vi "HFRR ADV v01.vi"() -> ()   [LabVIEW 2025] (continued)
            n2946 = case shown="False" w3205 {
              frame False {
                n2947 = disable-structure shown="Disabled" {
                  frame Disabled {
                    n2948 = stacked-sequence {
                      frame #0 {
                        n2949 = local write "RUN"(FALSE ("OK Button 2")) -> ()
                      }
                      frame #1 {
                      }
                    }
                  }
                  frame Enabled {
                  }
                }
              }
              frame True {
              }
            }
          }
        }
        n2950 = local read "Reset Graph"() -> (w3102:bool)
        n2951 = case shown="True" w3102 {
          selector: w3102 -> [_ w3119]
          frame False {
          }
          frame True {
            w3133 = 0.0 ("X Scale.Range:Maximum")
            n2952 = Not(x=w3119) -> (.not. x?=w3118:bool)
            n2953 = local write "Reset Graph"(w3118) -> ()
            n2954 = property on="Electrical Contact Resistance ( % )" class="WFChart (strict)"("XScale.Maximum"=600.0 ("X Scale.Range:Maximum"), "XScale.Minimum"=0.0 ("X Scale.Range:Minimum"), "YScale.Maximum"=100.0 ("Y Scale.Range:Maximum"), "YScale.Minimum"=0.0 ("Y Scale.Range:Minimum")) -> ()  [unwired: 2 in, 2 out]
            n2955 = property on="Frictional Force ( N )" class="WFChart (strict)"("XScale.Maximum"=600.0 ("X Scale.Range:Maximum"), "XScale.Minimum"=0.0 ("X Scale.Range:Minimum"), "YScale.Maximum"=100.0 ("Y Scale.Range:Maximum"), "YScale.Minimum"=0.0 ("Y Scale.Range:Minimum")) -> ()  [unwired: 2 in, 2 out]
            n2956 = property on="Temperature ( Deg C )" class="WFChart (strict)"("XScale.Maximum"=600.0 ("X Scale.Range:Maximum"), "XScale.Minimum"=0.0 ("X Scale.Range:Minimum"), "YScale.Maximum"=100.0 ("Y Scale.Range:Maximum"), "YScale.Minimum"=0.0 ("Y Scale.Range:Minimum")) -> ()  [unwired: 2 in, 2 out]
            n2957 = property on="Stroke ( mm )" class="WFChart (strict)"("XScale.Maximum"=600.0 ("X Scale.Range:Maximum"), "XScale.Minimum"=0.0 ("X Scale.Range:Minimum"), "YScale.Maximum"=100.0 ("Y Scale.Range:Maximum"), "YScale.Minimum"=0.0 ("Y Scale.Range:Minimum")) -> ()  [unwired: 2 in, 2 out]
            n2958 = property on="Coefficient of Friction" class="WFChart (strict)"("XScale.Maximum"=600.0 ("X Scale.Range:Maximum"), "XScale.Minimum"=0.0 ("X Scale.Range:Minimum"), "YScale.Maximum"=100.0 ("Y Scale.Range:Maximum"), "YScale.Minimum"=0.0 ("Y Scale.Range:Minimum")) -> ()  [unwired: 2 in, 2 out]
            n2959 = property on="Electrical Contact Resistance ( % )" class="WFChart (strict)"("XScale.Minimum"=0.0 ("X Scale.Range:Minimum"), "XScale.Maximum"=600.0 ("X Scale.Range:Maximum"), "YScale.Minimum"=0.0 ("Y Scale.Range:Minimum"), "YScale.Maximum"=100.0 ("Y Scale.Range:Maximum")) -> ()  [unwired: 2 in, 2 out]
            n2960 = property on="Temperature ( Deg C )" class="WFChart (strict)"("XScale.Minimum"=0.0 ("X Scale.Range:Minimum"), "XScale.Maximum"=600.0 ("X Scale.Range:Maximum"), "YScale.Minimum"=0.0 ("Y Scale.Range:Minimum"), "YScale.Maximum"=100.0 ("Y Scale.Range:Maximum")) -> ()  [unwired: 2 in, 2 out]
            n2961 = property on="Coefficient of Friction" class="WFChart (strict)"("XScale.Minimum"=0.0 ("X Scale.Range:Minimum"), "XScale.Maximum"=600.0 ("X Scale.Range:Maximum"), "YScale.Maximum"=1.0 ("X Scale.Range:Minimum"), "YScale.Minimum"=0.0 ("X Scale.Range:Minimum")) -> ()  [unwired: 2 in, 2 out]
            n2962 = property on="Frictional Force ( N )" class="WFChart (strict)"("XScale.Maximum"=600.0 ("X Scale.Range:Maximum"), "XScale.Minimum"=w3133, "YScale.Maximum"=10.0 ("Y Scale.Range:Maximum"), "YScale.Minimum"=w3133) -> ()  [unwired: 2 in, 2 out]
            n2963 = property on="Stroke ( mm )" class="WFChart (strict)"("XScale.Maximum"=600.0 ("X Scale.Range:Maximum"), "XScale.Minimum"=0.0 ("X Scale.Range:Minimum"), "YScale.Maximum"=100.0 ("Y Scale.Range:Maximum"), "YScale.Minimum"=0.0 ("Y Scale.Range:Minimum")) -> ()  [unwired: 2 in, 2 out]
          }
        }
      }
      frame "Compare Files" {
        # "Elapsed time\ncof\nstroke\nAir temp\nTemp\nHumidity"
        n2964 = case shown="True" "RSTV1 2" {
          frame False {
          }
          frame True {
            n2965 = property on="Humidity ( %RH )" class="XYGraph (strict)"("Y Scale.Display Format:Precision"=u8 0 ("Y Scale.Format & Precision:Precision")) -> ()  [unwired: 2 in, 2 out]
            n2966 = property on="Humidity ( %RH )" class="XYGraph (strict)"("X Scale.Range:Minimum"=0.0, "X Scale.Range:Maximum"=75.0, "Y Scale.Range:Minimum"=48.0, "Y Scale.Range:Maximum"=58.0) -> ()  [unwired: 2 in, 2 out]
          }
        }
        n2967 = case shown="True" "RST CP 2" {
          frame False {
          }
          frame True {
            n2968 = property on="XY Graph 13" class="XYGraph (strict)"("Y Scale.Display Format:Precision"=u8 0 ("Y Scale.Format & Precision:Precision")) -> ()  [unwired: 2 in, 2 out]
            n2969 = property on="XY Graph 13" class="XYGraph (strict)"("X Scale.Range:Minimum"=0.0, "X Scale.Range:Maximum"=75.0, "Y Scale.Range:Minimum"=0.0, "Y Scale.Range:Maximum"=100.0) -> ()  [unwired: 2 in, 2 out]
          }
        }
        n2970 = case shown="True" "RST CP" {
          frame False {
          }
          frame True {
            n2971 = property on="Sample Temperature ( °C )" class="XYGraph (strict)"("Y Scale.Display Format:Precision"=u8 2 ("Y Scale.Format & Precision:Precision")) -> ()  [unwired: 2 in, 2 out]
            n2972 = property on="Sample Temperature ( °C )" class="XYGraph (strict)"("X Scale.Range:Minimum"=0.0, "X Scale.Range:Maximum"=75.0, "Y Scale.Range:Minimum"=58.0, "Y Scale.Range:Maximum"=62.0) -> ()  [unwired: 2 in, 2 out]
          }
        }
        n2973 = case shown="True" "RSTV1 3" {
          frame False {
          }
          frame True {
            n2974 = property on="Air Temperature  ( °C )" class="XYGraph (strict)"("Y Scale.Display Format:Precision"=u8 2 ("Y Scale.Format & Precision:Precision")) -> ()  [unwired: 2 in, 2 out]
            n2975 = property on="Air Temperature  ( °C )" class="XYGraph (strict)"("X Scale.Range:Minimum"=0.0 ("Y Scale.Range:Minimum"), "X Scale.Range:Maximum"=75.0 ("Y Scale.Range:Maximum"), "Y Scale.Range:Minimum"=20.0 ("X Scale.Range:Minimum"), "Y Scale.Range:Maximum"=26.0 ("X Scale.Range:Maximum")) -> ()  [unwired: 2 in, 2 out]
          }
        }
        n2976 = case shown="True" "RSTV1 4" {
          frame False {
          }
          frame True {
            n2977 = property on="Stroke ( mm )" class="XYGraph (strict)"("Y Scale.Display Format:Precision"=u8 2 ("Y Scale.Format & Precision:Precision")) -> ()  [unwired: 2 in, 2 out]
            n2978 = property on="Stroke ( mm )" class="XYGraph (strict)"("X Scale.Range:Minimum"=0.0 ("Y Scale.Range:Maximum"), "X Scale.Range:Maximum"=75.0 ("X Scale.Range:Minimum"), "Y Scale.Range:Minimum"=0.98, "Y Scale.Range:Maximum"=1.02) -> ()  [unwired: 2 in, 2 out]
          }
        }
        n2979 = case shown="True" "rstv2" {
          frame False {
          }
          frame True {
            n2980 = property on="Coefficient Of Friction" class="XYGraph (strict)"("Y Scale.Display Format:Precision"=u8 3 ("Y Scale.Format & Precision:Precision")) -> ()  [unwired: 2 in, 2 out]
            n2981 = property on="Coefficient Of Friction" class="XYGraph (strict)"("X Scale.Range:Minimum"=0.0 ("Y Scale.Range:Maximum"), "X Scale.Range:Maximum"=75.0, "Y Scale.Range:Minimum"=0.0, "Y Scale.Range:Maximum"=1.0 ("X Scale.Range:Minimum")) -> ()  [unwired: 2 in, 2 out]
          }
        }
        n2982 = case shown="True" "RST CP 3" {
          frame False {
          }
          frame True {
            n2983 = property on="Air Temp ( °C ) vs Humidity ( % RH )" class="XYGraph (strict)"("X Scale.Range:Minimum"=18.0, "X Scale.Range:Maximum"=28.0 ("X Scale.Range:Minimum"), "Y Scale.Range:Minimum"=30.0 ("X Scale.Range:Minimum"), "Y Scale.Range:Maximum"=70.0 ("X Scale.Range:Minimum")) -> ()  [unwired: 2 in, 2 out]
          }
        }
        n2984 = case shown="True" "OPEN 1" {
          frame False {
          }
          frame True {
            (unwired) 0  # existing file
            w3775 = "Choose a datalog file to open"  # prompt
            n2985 = local write "OPEN 1"(FALSE ("OPEN 1")) -> ()
            n2986 = String To Path(string="C:\\LAB-IQ\\Data\\") -> (path=w3760:path)
            n2987 = File Dialog(6:"*.dgf" ("pattern"), 7:w3775, 11:w3760) -> (0:w3758:errorcluster, 3:w3766:path)  [unwired: 4 in, 2 out]
            n2988 = Unbundle(w3758) -> ()  [unwired: 3 out]
            n2989 = Strip Path(path=w3766) -> (name=w3765:string)  [unwired: 1 out]
            n2990 = Path To String(path=w3766) -> (string=w3761:string)
            "string1" <- w3761
            n2991 = Match Pattern(string=w3765, regular expression=".dgf") -> (before substring=→"String Control":string)  [unwired: 1 in, 3 out]
            n2992 = Match Pattern(string=w3761, regular expression=".dgf" ("substring (\"\")")) -> (before substring=w3771:string)  [unwired: 1 in, 3 out]
            n2993 = Concatenate Strings(w3771, ".duf" ("Substring")) -> (w3767:string)
            n2994 = String To Path(string=w3767) -> (path=w3772:path)
            n2995 = call <vilib>:"Read Characters From File.vi"("file path (dialog if empty)"=w3772, "start of read offset (chars.:0)"=60 ("start of read offset (chars.: 0)")) -> ("character string"=→"String Control 2":string)  [unwired: 4 in, 3 out]
          }
        }
        n2996 = case shown="True" "OPEN 2" {
          frame False {
          }
          frame True {
            (unwired) 0  # existing file
            w3793 = "Choose a datalog file to open"  # prompt
            n2997 = local write "OPEN 2"(FALSE ("OPEN 1")) -> ()
            n2998 = String To Path(string="C:\\LAB-IQ\\Data\\") -> (path=w3778:path)
            n2999 = File Dialog(6:"*.dgf" ("pattern"), 7:w3793, 11:w3778) -> (0:w3776:errorcluster, 3:w3784:path)  [unwired: 4 in, 2 out]
            n3000 = Unbundle(w3776) -> ()  [unwired: 3 out]
            n3001 = Strip Path(path=w3784) -> (name=w3782:string)  [unwired: 1 out]
            n3002 = Path To String(path=w3784) -> (string=w3779:string)
            "string1 2" <- w3779
            n3003 = Match Pattern(string=w3782, regular expression=".dgf") -> (before substring=→"String Control 3":string)  [unwired: 1 in, 3 out]
            n3004 = Match Pattern(string=w3779, regular expression=".dgf" ("substring (\"\")")) -> (before substring=w3790:string)  [unwired: 1 in, 3 out]
            n3005 = Concatenate Strings(w3790, ".duf" ("Substring")) -> (w3787:string)
            n3006 = String To Path(string=w3787) -> (path=w3785:path)
            n3007 = call <vilib>:"Read Characters From File.vi"("file path (dialog if empty)"=w3785, "start of read offset (chars.:0)"=60 ("start of read offset (chars.: 0)")) -> ("character string"=→"String Control 4":string)  [unwired: 4 in, 3 out]
          }
        }
        n3008 = case shown="True" "OPEN 3" {
          frame False {
          }
          frame True {
            (unwired) 0  # existing file
            w3811 = "Choose a datalog file to open"  # prompt
            n3009 = local write "OPEN 3"(FALSE ("OPEN 1")) -> ()
            n3010 = String To Path(string="C:\\LAB-IQ\\Data\\") -> (path=w3796:path)
            n3011 = File Dialog(6:"*.dgf" ("pattern"), 7:w3811, 11:w3796) -> (0:w3794:errorcluster, 3:w3802:path)  [unwired: 4 in, 2 out]
            n3012 = Unbundle(w3794) -> ()  [unwired: 3 out]
            n3013 = Strip Path(path=w3802) -> (name=w3800:string)  [unwired: 1 out]
            n3014 = Path To String(path=w3802) -> (string=w3797:string)
            "string1 3" <- w3797
            n3015 = Match Pattern(string=w3800, regular expression=".dgf") -> (before substring=→"String Control 5":string)  [unwired: 1 in, 3 out]
            n3016 = Match Pattern(string=w3797, regular expression=".dgf" ("substring (\"\")")) -> (before substring=w3807:string)  [unwired: 1 in, 3 out]
            n3017 = Concatenate Strings(w3807, ".duf" ("Substring")) -> (w3804:string)
            n3018 = String To Path(string=w3804) -> (path=w3808:path)
            n3019 = call <vilib>:"Read Characters From File.vi"("file path (dialog if empty)"=w3808, "start of read offset (chars.:0)"=60 ("start of read offset (chars.: 0)")) -> ("character string"=→"String Control 6":string)  [unwired: 4 in, 3 out]
          }
        }
        n3020 = case shown="True" "OPEN 4" {
          frame False {
          }
          frame True {
            (unwired) 0  # existing file
            w3829 = "Choose a datalog file to open"  # prompt
            n3021 = local write "OPEN 4"(FALSE ("OPEN 1")) -> ()
            n3022 = String To Path(string="C:\\LAB-IQ\\Data\\") -> (path=w3814:path)
            n3023 = File Dialog(6:"*.dgf" ("pattern"), 7:w3829, 11:w3814) -> (0:w3812:errorcluster, 3:w3820:path)  [unwired: 4 in, 2 out]
            n3024 = Unbundle(w3812) -> ()  [unwired: 3 out]
            n3025 = Strip Path(path=w3820) -> (name=w3818:string)  [unwired: 1 out]
            n3026 = Path To String(path=w3820) -> (string=w3815:string)
            "string1 4" <- w3815
            n3027 = Match Pattern(string=w3818, regular expression=".dgf") -> (before substring=→"String Control 7":string)  [unwired: 1 in, 3 out]
            n3028 = Match Pattern(string=w3815, regular expression=".dgf" ("substring (\"\")")) -> (before substring=w3825:string)  [unwired: 1 in, 3 out]
            n3029 = Concatenate Strings(w3825, ".duf" ("Substring")) -> (w3822:string)
            n3030 = String To Path(string=w3822) -> (path=w3826:path)
            n3031 = call <vilib>:"Read Characters From File.vi"("file path (dialog if empty)"=w3826, "start of read offset (chars.:0)"=60 ("start of read offset (chars.: 0)")) -> ("character string"=→"String Control 8":string)  [unwired: 4 in, 3 out]
          }
        }
      }
      frame "About" {
        # "Elapsed time\ncof\nstroke\nmean pos\nTemp\nHumidity"
        n3032 = disable-structure shown="Disabled" {
          frame Disabled {
            n3033 = case shown="True" "Export" {
              frame False {
              }
              frame True {
                w3851 = "                                      " ("string")
                w3853 = "\r"
                (unwired) i16 6 ("width (-)")
                w3930 = "\r"
                w3862 = "\r"
                n3034 = local write "Export"(FALSE ("Export")) -> ()
                n3035 = local read "String 29"() -> (w3899:string)
                n3036 = local read "String 34"() -> (w3887:string)
                n3037 = local read "String 35"() -> (w3882:string)
                n3038 = local read "String 37"() -> (w3878:string)
                n3039 = local read "String 36"() -> (w3875:string)
                n3040 = local read "String 38"() -> (w3872:string)
                n3041 = local read "String 39"() -> (w3869:string)
                n3042 = Match Pattern(string=w3899, regular expression=".dwm") -> (before substring=w3895:string)  [unwired: 1 in, 3 out]
                "before substring" <- w3895
                n3043 = local read "S 38"() -> (w3890:string)
                n3044 = local read "S 39"() -> (w3883:string)
                n3045 = local read "Temperature before test 2"() -> (w3919:dbl)
                n3046 = local read "Temperature after test 2"() -> (w3924:dbl)
                n3047 = local read "Humidity before test 2"() -> (w3905:dbl)
                n3048 = local read "Humidity after test 2"() -> (w3920:dbl)
                n3049 = local read "MWSD 2"() -> (w3916:dbl)
                n3050 = local read "WS1.4 2"() -> (w3932:dbl)
                n3051 = local read "HCF 2"() -> (w3928:dbl)
                n3052 = local read "AVP 2"() -> (w3917:dbl)
                n3053 = Concatenate Strings("1," ("string"), w3890) -> (w3889:string)
                n3054 = Concatenate Strings("2," ("string"), w3887) -> (w3886:string)
                n3055 = Concatenate Strings("3," ("string"), w3883) -> (w3885:string)
                n3056 = Concatenate Strings("4," ("string"), w3882) -> (w3881:string)
                n3057 = Concatenate Strings("5," ("string"), w3878) -> (w3879:string)
                n3058 = Concatenate Strings("6," ("string"), w3875) -> (w3876:string)
                n3059 = Concatenate Strings("7," ("string"), w3872) -> (w3873:string)
                n3060 = Concatenate Strings("8," ("string"), w3869) -> (w3870:string)
                n3061 = local read "Sample ID"() -> (w3937:string)
                n3062 = case shown="\"xlx\"" "Select File Type" {
                  tunnel: w3895 -> [w3940 w3942 w3944]
                  tunnel: [w3938 w3943 w3945] -> w3894
                  frame "xlx" {
                    n3063 = Concatenate Strings(w3940, ".xls" ("string")) -> (w3938:string)
                  }
                  frame "csv" {
                    n3064 = Concatenate Strings(w3942, ".csv" ("string")) -> (w3943:string)
                  }
                  frame "txt" {
                    n3065 = Concatenate Strings(w3944, ".txt" ("string")) -> (w3945:string)
                  }
                }
                n3066 = local read "Test Date"() -> (w3936:string)
                n3067 = local read "String 45"() -> (w3850:string)
                n3068 = local read "String 31"() -> (w3935:string)
                n3069 = local read "String 32"() -> (w3934:string)
                n3070 = local read "TITTLE"() -> (w3858:string)
                n3071 = Number To Fractional String(number=w3905, width (-)=i16 6, precision (6)=i16 2) -> (F-format string=w3904:string)  [unwired: 1 in]
                n3072 = Number To Fractional String(number=w3919, width (-)=i16 6, precision (6)=i16 2) -> (F-format string=w3925:string)  [unwired: 1 in]
                n3073 = Number To Fractional String(number=w3920, width (-)=i16 6, precision (6)=i16 2) -> (F-format string=w3918:string)  [unwired: 1 in]
                n3074 = Number To Fractional String(number=w3924, width (-)=i16 6, precision (6)=i16 2) -> (F-format string=w3923:string)  [unwired: 1 in]
                n3075 = Number To Fractional String(number=w3916, width (-)=i16 6, precision (6)=i16 2) -> (F-format string=w3914:string)  [unwired: 1 in]
                n3076 = Number To Fractional String(number=w3917, width (-)=i16 6, precision (6)=i16 2) -> (F-format string=w3915:string)  [unwired: 1 in]
                n3077 = Number To Fractional String(number=w3928, width (-)=i16 6, precision (6)=i16 2) -> (F-format string=w3929:string)  [unwired: 1 in]
                n3078 = Number To Fractional String(number=w3932, precision (6)=i16 2) -> (F-format string=w3933:string)  [unwired: 2 in]
                n3079 = local read "s.NO"() -> (w3852:string)
                n3080 = Concatenate Strings("=" ("string"), w3858) -> (w3857:string)
                n3081 = Concatenate Strings("S.No," ("string"), "                                       Parameters" ("string")) -> (w3863:string)
                n3082 = Concatenate Strings(w3930, w3889, w3904, w3930, w3886, w3925, w3930, w3885, w3918, w3930, w3881, w3923, w3930, w3879, w3914, w3930, w3876, w3915, w3930, w3873, w3929, w3930, w3870, w3933) -> (w3892:string)
                n3083 = Concatenate Strings(w3862, "," ("string"), w3850, w3852, w3851, w3934, w3937, w3851, w3935, w3936, w3862) -> (w3860:string)
                n3084 = local read "Tested by"() -> (w3866:string)
                n3085 = local read "String 33"() -> (w3867:string)
                n3086 = Concatenate Strings("," ("string"), "                                                                             " ("string")) -> (w3855:string)
                n3087 = Concatenate Strings(w3857, w3853, w3860, w3853, w3863, w3892, w3853, w3855, w3867, w3866) -> (→"export":string)
                n3088 = String To Path(string=w3894) -> (path=w3901:path)
                n3089 = local read "export"() -> (w3896:string)
                n3090 = call <vilib>:"Write Characters To File.vi"("append to file? (new file:F)"=FALSE, "character string"=w3896, "file path (dialog if empty)"=w3901) -> ()  [unwired: 2 in, 1 out]
              }
            }
          }
          frame Enabled {
          }
        }
        n3091 = case shown="True" "OK Button 17" {
          frame False {
          }
          frame True {
            (unwired) 0  # existing file
            w4154 = "Choose a datalog file to open"  # prompt
            n3092 = local write "OK Button 17"(FALSE ("OK Button 17")) -> ()
            n3093 = local read "String"() -> (w4149:string)
            n3094 = String To Path(string=w4149) -> (path=w4150:path)
            n3095 = File Dialog(6:"*.duf" ("pattern"), 7:w4154, 11:w4150) -> (0:w4141:errorcluster, 3:w4160:path)  [unwired: 4 in, 2 out]
            n3096 = Unbundle(w4141) -> ()  [unwired: 3 out]
            n3097 = Open/Create/Replace File "Open File"(file path (use dialog)=w4160) -> (refnum out=w4152:refnum<file>)  [unwired: 5 in, 2 out]
            n3098 = Strip Path(path=w4160) -> (name=w4158:string)  [unwired: 1 out]
            n3099 = Path To String(path=w4160) -> (string=w4143:string)
            n3100 = while {
              tunnel: w4152 -> [w4164]
              i -> [w4161]
              stop <- w4162 continue-if-true
              (unwired) TRUE ("line mode (F)")
              n3101 = Read from Text File "Read File"(file (use dialog)=w4164) -> (text=w4163:string)  [unwired: 3 in, 3 out]
              n3102 = local write "Numeric 16"(w4161) -> ()
              n3103 = String Length(string=w4163) -> (length=w4166:i32)
              n3104 = Greater?(x=w4166, y=1) -> (0:w4162:bool)
            }
            n3105 = local write "String 29"(w4143) -> ()
            n3106 = Search and Replace String(input string=w4143, search string=".duf", replace string=".dgf" ("replace string (\"\")")) -> (result string=→"String Indicator 4":string)  [unwired: 5 in, 3 out]
            n3107 = Match Pattern(string=w4158, regular expression=".dwm") -> (before substring=w4142:string)  [unwired: 1 in, 3 out]
            "String Indicator" <- w4142
            n3108 = Match Pattern(string=w4143, regular expression=".dwm" ("substring (\"\")")) -> (before substring=w4144:string)  [unwired: 1 in, 3 out]
            "String Indicator 3" <- w4144
            n3109 = local write "TITTLE 2"(w4142) -> ()
            n3110 = String To Path(string=w4144) -> (path=w4151:path)
            "path" <- w4151
            n3111 = call <vilib>:"Read Characters From File.vi"("file path (dialog if empty)"=w4151, "start of read offset (chars.:0)"=60 ("start of read offset (chars.: 0)")) -> ("character string"=→"String Indicator 2":string)  [unwired: 4 in, 3 out]
          }
        }
        n3112 = call <vilib>:"Query Available Printers.vi"() -> ("system configured printers"=w3843:string[])  [unwired: 9 in, 2 out]
        "System Configured Printers 2" <- w3843
        n3113 = local read "OK Button 16"() -> (w3840:bool)
        n3114 = case shown="True" "OK Button 16" {
          frame False {
          }
          frame True {
            n3115 = stacked-sequence {
              frame #0 {
                n3116 = local read "Numeric 16"() -> (w4168:i32)
                n3117 = local write "Numeric 10"(w4168) -> ()
              }
              frame #1 {
                n3118 = local read "String 29"() -> (w4171:string)
                n3119 = String To Path(string=w4171) -> (path=w4170:path)
                n3120 = Open/Create/Replace File "Open File"(file path (use dialog)=w4170) -> (refnum out=w4172:refnum<file>)  [unwired: 5 in, 2 out]
                n3121 = for {
                  N: 16 -> [_]
                  tunnel: w4172 -> [w4179]
                  i -> [w4175]
                  (unwired) TRUE ("line mode (F)")
                  n3122 = Read from Text File "Read File"(file (use dialog)=w4179) -> (text=w4173:string)  [unwired: 3 in, 3 out]
                  n3123 = Match Pattern(string=w4173, regular expression="(") -> (after substring=w4178:string)  [unwired: 1 in, 3 out]
                  n3124 = Match Pattern(string=w4178, regular expression=")") -> (before substring=w4174:string)  [unwired: 1 in, 3 out]
                  n3125 = case shown="1" w4175 {
                    tunnel: w4174 -> [w4180 w4181 _ _ w4182 w4183 w4184 w4186 w4188 w4190 w4192 w4194 w4196 w4198 _]
                    tunnel: w4173 -> [_ _ _ _ _ _ _ _ _ _ _ _ _ _ _]
                    frame 0 {
                      "TITTLE" <- w4180
                    }
                    frame 1 {
                      "Sample ID" <- w4181
                    }
                    frame 2 {
                    }
                    frame 3 {
                    }
                    frame 4 {
                      "Test Date" <- w4182
                    }
                    frame 5 {
                      "Tested by" <- w4183
                    }
                    frame 6 {
                      n3126 = Fract/Exp String To Number(string=w4184) -> (number=→"Humidity before test 2":dbl)  [unwired: 3 in, 1 out]
                    }
                    frame 7 {
                      n3127 = Fract/Exp String To Number(string=w4186) -> (number=→"Temperature before test 2":dbl)  [unwired: 3 in, 1 out]
                    }
                    frame 8 {
                      n3128 = Fract/Exp String To Number(string=w4188) -> (number=→"Humidity after test 2":dbl)  [unwired: 3 in, 1 out]
                    }
                    frame 9 {
                      n3129 = Fract/Exp String To Number(string=w4190) -> (number=→"Temperature after test 2":dbl)  [unwired: 3 in, 1 out]
                    }
                    frame 10 {
                      n3130 = Fract/Exp String To Number(string=w4192) -> (number=→"MWSD 2":dbl)  [unwired: 3 in, 1 out]
                    }
                    frame 11 {
                      n3131 = Fract/Exp String To Number(string=w4194) -> (number=→"AVP 2":dbl)  [unwired: 3 in, 1 out]
                    }
                    frame 12 {
                      n3132 = Fract/Exp String To Number(string=w4196) -> (number=→"HCF 2":dbl)  [unwired: 3 in, 1 out]
                    }
                    frame 13 {
                      n3133 = Fract/Exp String To Number(string=w4198) -> (number=→"WS1.4 2":dbl)  [unwired: 3 in, 1 out]
                    }
                    frame 14, Default {
                    }
                  }
                }
              }
              frame #2 {
              }
            }
            n3134 = local write "OK Button 16"(FALSE ("OK Button 13")) -> ()
          }
        }
        n3135 = Index Array(array=w3843, index="Select Printer 3") -> (element=w3845:string)
        "Selected Printer" <- w3845
        n3136 = case shown="True" w3840 {
          frame False {
          }
          frame True {
            n3137 = flat-sequence {
              frame #0 {
              }
              frame #1 {
                n3138 = Wait (ms)(milliseconds to wait=u32 100) -> ()  [unwired: 1 out]
              }
              frame #2 {
                n3139 = local write "OK Button 16"(FALSE ("Print 3")) -> ()
              }
            }
          }
        }
        n3140 = case shown="True" "Print" {
          tunnel: w3845 -> [_ w4137]
          frame False {
          }
          frame True {
            (unwired) i16 6 ("width (-)")
            (unwired) "TESTED BY : "
            (unwired) "TESTED DATE :"
            (unwired) "SAMPLE ID : "
            (unwired) "SAMPLE DESIGN : "
            w4095 = "\r"
            w4112 = "\r"
            # "add image"
            n3141 = local read "Sample ID"() -> (w4085:string)
            n3142 = local read "Tested by"() -> (w4088:string)
            n3143 = local read "String 34"() -> (w4075:string)
            n3144 = local read "String 45"() -> (w4055:string)
            n3145 = local read "String 35"() -> (w4070:string)
            n3146 = local read "String 37"() -> (w4068:string)
            n3147 = local read "String 32"() -> (w4090:string)
            n3148 = local read "String 36"() -> (w4065:string)
            n3149 = local read "String 31"() -> (w4089:string)
            n3150 = local read "Test Date"() -> (w4086:string)
            n3151 = local read "String 33"() -> (w4091:string)
            n3152 = local read "String 38"() -> (w4061:string)
            n3153 = local read "String 39"() -> (w4058:string)
            n3154 = local write "Print"(FALSE ("Print FF")) -> ()
            n3155 = local read "S 39"() -> (w4073:string)
            n3156 = local read "S 38"() -> (w4080:string)
            n3157 = local read "Temperature before test 2"() -> (w4111:dbl)
            n3158 = local read "Temperature after test 2"() -> (w4101:dbl)
            n3159 = local read "Humidity before test 2"() -> (w4126:dbl)
            n3160 = local read "Humidity after test 2"() -> (w4110:dbl)
            n3161 = local read "MWSD 2"() -> (w4115:dbl)
            n3162 = local read "WS1.4 2"() -> (w4093:dbl)
            n3163 = Concatenate Strings("2)" ("string"), w4075) -> (w4076:string)
            n3164 = Concatenate Strings("3)" ("string"), w4073) -> (w4074:string)
            n3165 = Concatenate Strings("1)" ("string"), w4080) -> (w4079:string)
            n3166 = Concatenate Strings("4)" ("string"), w4070) -> (w4071:string)
            n3167 = Concatenate Strings("5)" ("string"), w4068) -> (w4067:string)
            n3168 = Concatenate Strings("6)" ("string"), w4065) -> (w4064:string)
            n3169 = Concatenate Strings("7)" ("string"), w4061) -> (w4062:string)
            n3170 = Concatenate Strings("8)" ("string"), w4058) -> (w4059:string)
            n3171 = local read "HCF 2"() -> (w4097:dbl)
            n3172 = local read "AVP 2"() -> (w4114:dbl)
            n3173 = local read "s.NO"() -> (w4056:string)
            n3174 = call <vilib>:"New Report.vi"("report type"=enum16{"Standard Report", "HTML"}."Standard Report") -> ("report out"=w4135:refnum<class "NI_report.lvclass">, "error out"=w4134:errorcluster)  [unwired: 13 in]
            n3175 = local read "TITTLE"() -> (w4087:string)
            n3176 = Concatenate Strings(w4112, w4055, w4056, w4112, w4090, w4085, w4112, w4089, w4086, w4112, w4091, w4088, w4112) -> (w4105:string)
            "test by" <- w4105
            n3177 = Number To Fractional String(number=w4111, width (-)=i16 6, precision (6)=i16 2) -> (F-format string=w4100:string)  [unwired: 1 in]
            n3178 = Number To Fractional String(number=w4110, width (-)=i16 6, precision (6)=i16 2) -> (F-format string=w4113:string)  [unwired: 1 in]
            n3179 = Number To Fractional String(number=w4126, width (-)=i16 6, precision (6)=i16 2) -> (F-format string=w4131:string)  [unwired: 1 in]
            n3180 = Number To Fractional String(number=w4115, width (-)=i16 6, precision (6)=i16 2) -> (F-format string=w4117:string)  [unwired: 1 in]
            n3181 = Number To Fractional String(number=w4101, width (-)=i16 6, precision (6)=i16 2) -> (F-format string=w4102:string)  [unwired: 1 in]
            n3182 = Number To Fractional String(number=w4114, width (-)=i16 6, precision (6)=i16 2) -> (F-format string=w4116:string)  [unwired: 1 in]
            n3183 = Number To Fractional String(number=w4097, width (-)=i16 6, precision (6)=i16 2) -> (F-format string=w4096:string)  [unwired: 1 in]
            n3184 = Number To Fractional String(number=w4093, precision (6)=i16 2) -> (F-format string=w4092:string)  [unwired: 2 in]
            n3185 = call-dynamic "Set Report Header Text.vi"("report in"=w4135, "center header text"=w4087, "error in (no error)"=w4134) -> ("report out"=w4106:refnum<class "NI_report.lvclass">, "error out"=w4107:errorcluster)  [unwired: 11 in]
            n3186 = Concatenate Strings(w4095, w4079, w4131, w4095, w4076, w4100, w4095, w4074, w4113, w4095, w4071, w4102, w4095, w4067, w4117, w4095, w4064, w4116, w4095, w4062, w4096, w4095, w4059, w4092) -> (w4083:string)
            "export 2" <- w4083
            n3187 = call-poly <vilib>:"Append Report Text.vi"("report in"=w4106, "text"=w4105, "error in (no error)"=w4107) -> ("report out"=w4109:refnum<class "NI_report.lvclass">, "error out"=w4108:errorcluster)  [unwired: 9 in, 2 out]
            n3188 = local read "test by"() -> (w4082:string)
            n3189 = local read "TITTLE"() -> (w4084:string)
            n3190 = call-poly <vilib>:"Append Report Text.vi"("report in"=w4109, "error in (no error)"=w4108) -> ("report out"=w4130:refnum<class "NI_report.lvclass">, "error out"=w4128:errorcluster)  [unwired: 10 in, 2 out]
            n3191 = Concatenate Strings(w4084, w4083, w4082) -> (→"output":string)
            n3192 = call-poly <vilib>:"Append Report Text.vi"("report in"=w4130, "text"=w4083, "error in (no error)"=w4128) -> ("report out"=w4129:refnum<class "NI_report.lvclass">, "error out"=w4127:errorcluster)  [unwired: 9 in, 2 out]
            n3193 = call-dynamic "Print Report.vi"("report in"=w4129, "printer name (default)"=w4137, "error in (no error)"=w4127) -> ("report out"=w4139:refnum<class "NI_report.lvclass">, "error out"=w4140:errorcluster)  [unwired: 11 in]
            n3194 = call-dynamic "Dispose Report.vi"("report in"=w4139, "error in (no error)"=w4140) -> ()  [unwired: 13 in, 1 out]
          }
        }
        n3195 = case shown="True" "Print 2" {
          frame False {
          }
          frame True {
            n3196 = flat-sequence {
              frame #0 {
                n3197 = local read "s.NO"() -> (→"s.NO 2":string)
                n3198 = Wait (ms)(milliseconds to wait=u32 20) -> ()  [unwired: 1 out]
                n3199 = local read "Sample ID  3"() -> (→"Sample ID  6":string)
                n3200 = local read "Sample ID  4"() -> (→"Sample ID  7":string)
                n3201 = local read "Sample ID"() -> (→"Sample ID  2":string)
                n3202 = local read "Tested by"() -> (→"Tested by 2":string)
                n3203 = local read "Test Date"() -> (→"Test Date 2":string)
                n3204 = local read "Humidity after test 3"() -> (→"Humidity after test 4":dbl)
                n3205 = local read "Ref A Test Date :"() -> (→"TITTLE 4":string)
                n3206 = local read "Temperature before test 3"() -> (w3962:dbl)
                n3207 = local read "Temperature before test 3"() -> (→"Temperature after test 5":dbl)
                n3208 = local read "Temperature after test 3"() -> (→"Temperature after test 4":dbl)
                n3209 = local read "Humidity before test 3"() -> (→"Humidity before test 4":dbl)
                n3210 = local write "Temperature before test 3"(w3962) -> ()
                n3211 = local read "image data"() -> (w3953:T2)
                n3212 = String To Path(string="C:\\LAB-IQ\\im\\Temp_resized.jpg") -> (path=w3954:path)
                "path 2" <- w3954
                n3213 = call <vilib>:"Write JPEG File.vi"("image data"=w3953, "path to JPEG file"=w3954) -> ()  [unwired: 8 in, 2 out]
                "Ref A Test Date :" <- "Ref A Test Date :"
                "Ref B Test Date :" <- "Ref B Test Date :"
                "Ref B Scar Value :" <- "Ref B Scar Value :"
                "Ref A Scar Value :" <- "Ref A Scar Value :"
              }
              frame #1 {
                (unwired) HTML_Report_Image_Alignment."MIDDLE" ("alignment (default)")
                w3990 = u16 0 items=["portrait", "landscape"] ("orientation (portrait)")
                (unwired) HTML_Report_Image_Alignment."ABSMIDDLE" ("alignment (default)")
                (unwired) "TESTED BY : "
                (unwired) "TESTED DATE :"
                (unwired) "SAMPLE ID : "
                (unwired) "SAMPLE DESIGN : "
                w4023 = "\r"
                # "add image"
                n3214 = Wait (ms)(milliseconds to wait=u32 20) -> ()  [unwired: 1 out]
                n3215 = local read "Sample ID  2"() -> (w4016:string)
                n3216 = local read "Wear Scar X"() -> (w3988:dbl)
                "Length ( microns ) 2" <- w3988
                n3217 = local read "Wear Scar Y"() -> (w3987:dbl)
                "Wear Scar Y ( microns ) :" <- w3987
                n3218 = local read "Test Date 2"() -> (w4017:string)
                n3219 = local read "Tested by 2"() -> (w4018:string)
                n3220 = local read "String 46"() -> (w4014:string)
                n3221 = local read "String 48"() -> (w4020:string)
                n3222 = local read "String 47"() -> (w4019:string)
                n3223 = local read "String 49"() -> (w4021:string)
                n3224 = local read "String 10"() -> (w3974:string)
                n3225 = local read "s.NO 2"() -> (w4015:string)
                n3226 = Add(x=w3988, y=w3987) -> (x+y=w3986:dbl)
                n3227 = call <vilib>:"New Report.vi"("report type"=enum16{"Standard Report", "HTML"}."HTML") -> ("report out"=w3994:refnum<class "NI_report.lvclass">, "error out"=w3992:errorcluster)  [unwired: 13 in]
                n3228 = Concatenate Strings(w4023, w4014, w4015, w4023, w4020, w4016, w4023, w4019, w4017, w4023, w4021, w4018, w4023) -> (→"test by 2":string)
                n3229 = Concatenate Strings("C:\\LAB-IQ\\Data\\" ("string"), w3974, ".jpg" ("string")) -> ()  [unwired: 1 out]
                n3230 = Divide(x=w3986, y=2.0) -> (x/y=→"Mean Wear ( microns) :":dbl)
                n3231 = call-dynamic "Set Report Orientation.vi"("report in"=w3994, "orientation (portrait)"=w3990, "error in (no error)"=w3992) -> ("report out"=w3993:refnum<class "NI_report.lvclass">, "error out"=w3991:errorcluster)  [unwired: 11 in]
                n3232 = for {
                  N: 5 -> [_]
                  tunnel: w3993 -> [w4044]
                  tunnel: [w4043] -> w3972
                  tunnel: w3991 -> [w4042]
                  tunnel: [w4041] -> w3971
                  n3233 = call-dynamic "Set Report Tab Width.vi"("report in"=w4044, "error in (no error)"=w4042) -> ("report out"=w4043:refnum<class "NI_report.lvclass">, "error out"=w4041:errorcluster)  [unwired: 12 in]
                }
                n3234 = local read "TITTLE"() -> (w3989:string)
                n3235 = call-dynamic "Set Report Header Text.vi"("report in"=w3972, "center header text"=w3989, "error in (no error)"=w3971) -> ("report out"=w4010:refnum<class "NI_report.lvclass">, "error out"=w4009:errorcluster)  [unwired: 11 in]
                n3236 = for {
                  N: 1 -> [_]
                  tunnel: [w4048] -> w3996
                  tunnel: [w4047] -> w3995
                  tunnel: w4010 -> [w4046]
                  tunnel: w4009 -> [w4045]
                  n3237 = call-dynamic "New Report Line.vi"("report in"=w4046, "error in (no error)"=w4045) -> ("report out"=w4048:refnum<class "NI_report.lvclass">, "error out"=w4047:errorcluster)  [unwired: 12 in]
                }
                n3238 = for {
                  N: 2 -> [_]
                  tunnel: [w4040] -> w4002
                  tunnel: [w4039] -> w4001
                  tunnel: w3996 -> [w4038]
                  tunnel: w3995 -> [w4037]
                  n3239 = call-dynamic "New Report Line.vi"("report in"=w4038, "error in (no error)"=w4037) -> ("report out"=w4040:refnum<class "NI_report.lvclass">, "error out"=w4039:errorcluster)  [unwired: 12 in]
                }
                n3240 = for {
                  N: 25 -> [_]
                  tunnel: w4002 -> [w4036]
                  tunnel: w4001 -> [w4034]
                  tunnel: [w4035] -> w4005
                  tunnel: [w4033] -> w4004
                  n3241 = call-dynamic "Set Report Tab Width.vi"("report in"=w4036, "error in (no error)"=w4034) -> ("report out"=w4035:refnum<class "NI_report.lvclass">, "error out"=w4033:errorcluster)  [unwired: 12 in]
                }
                n3242 = control-ref of="Tab Control 9"() -> (w4000:refnum<vi>)
                n3243 = call-dynamic "Append Control Image to Report.vi"("report in"=w4005, "alignment (default)"=HTML_Report_Image_Alignment."ABSMIDDLE", "ctrl reference"=w4000, "error in (no error)"=w4004) -> ("report out"=w3999:refnum<class "NI_report.lvclass">, "error out"=w3998:errorcluster)  [unwired: 8 in, 2 out]
                n3244 = for {
                  N: 3 -> [_]
                  tunnel: [w4032] -> w3983
                  tunnel: [w4031] -> w3982
                  tunnel: w3999 -> [w4030]
                  tunnel: w3998 -> [w4029]
                  n3245 = call-dynamic "New Report Line.vi"("report in"=w4030, "error in (no error)"=w4029) -> ("report out"=w4032:refnum<class "NI_report.lvclass">, "error out"=w4031:errorcluster)  [unwired: 12 in]
                }
                n3246 = for {
                  N: 100 -> [_]
                  tunnel: w3983 -> [w4028]
                  tunnel: w3982 -> [w4026]
                  tunnel: [w4027] -> w3979
                  tunnel: [w4025] -> w3977
                  n3247 = call-dynamic "Set Report Tab Width.vi"("report in"=w4028, "error in (no error)"=w4026) -> ("report out"=w4027:refnum<class "NI_report.lvclass">, "error out"=w4025:errorcluster)  [unwired: 12 in]
                }
                n3248 = String To Path(string="C:\\LAB-IQ\\im\\Temp_resized.jpg") -> (path=w3969:path)
                n3249 = call-poly <vilib>:"Append Image to Report.vi"("report in"=w3979, "path or URL of image"=w3969, "error in (no error)"=w3977) -> ("report out"=w3978:refnum<class "NI_report.lvclass">, "error out"=w3976:errorcluster)  [unwired: 9 in, 2 out]
                n3250 = call-poly <vilib>:"Open HTML Report in Browser.vi"("report in"=w3978, "error in (no error)"=w3976) -> ("report out"=w4013:refnum<class "NI_report.lvclass">, "error out"=w4012:errorcluster)  [unwired: 11 in, 1 out]
                n3251 = call-dynamic "Dispose Report.vi"("report in"=w4013, "error in (no error)"=w4012) -> ()  [unwired: 13 in, 1 out]
              }
              frame #2 {
              }
              frame #3 {
                n3252 = disable-structure shown="Disabled" {
                  frame Disabled {
                    n3253 = local read "String 10"() -> (w4053:string)
                    n3254 = Concatenate Strings("C:\\LAB-IQ-NXT\\Data\\" ("string"), w4053, ".jpg" ("string")) -> (w4051:string)
                    n3255 = String To Path(string=w4051) -> (path=w4050:path)
                    n3256 = Delete(path (use dialog)=w4050) -> ()  [unwired: 4 in, 3 out]
                  }
                  frame Enabled {
                  }
                }
                n3257 = local write "Print 2"(FALSE ("Print")) -> ()
              }
            }
          }
        }
      }
    }
    n3258 = Wait (ms)(milliseconds to wait=u32 50) -> ()  [unwired: 1 out]
    n3259 = Wait (ms)(milliseconds to wait=u32 50) -> ()  [unwired: 1 out]
    n3260 = local read "Quit"() -> (w2395:bool)
  }
  n3261 = VISA Close(VISA resource name=w46, error in (no error)=w45) -> ()  [unwired: 1 out]
  n3262 = while {
    stop <- w4204 stop-if-true
    n3263 = local read "Auto Start Test"() -> (w4202:bool)
    n3264 = local read "RUN"() -> (w4201:bool)
    n3265 = Wait (ms)(milliseconds to wait=u32 1000) -> ()  [unwired: 1 out]
    n3266 = Or(x=w4201, y=w4202) -> (x .or. y?=w4200:bool)
    n3267 = case shown="True" w4200 {
      frame False {
      }
      frame True {
        n3268 = local read "LVDT STROKE Actual"() -> (w4205:dbl)
        n3269 = In Range and Coerce(upper limit=1.2, x=w4205, lower limit=0.6) -> (In Range?=w4208:bool)  [unwired: 1 out]
        n3270 = call-poly <vilib>:"Random Number (Range).vi"("lower bound (0)"=0.998 ("upper bound (100)"), "upper bound (100)"=1.003) -> ("number"=w4206:dbl)  [unwired: 9 in]
        n3271 = case shown="True" w4208 {
          tunnel: [w4213 w4214] -> w4207
          tunnel: w4206 -> [_ w4214]
          tunnel: w4205 -> [w4213 _]
          frame False {
          }
          frame True {
          }
        }
        "LVDT STROKE DISPLAY" <- w4207
      }
    }
    n3272 = local read "Quit"() -> (w4204:bool)
  }
  n3273 = while {
    tunnel: [w4231] -> w54
    shift-right: [w4224] -> _
    shift-left: 0.0 -> [w4227]
    shift-right: [w4223] -> _
    shift-left: 0.0 -> [w4226]
    shift-right: [w4222] -> _
    shift-left: 100.0 ("vc_cmd") -> [w4225]
    stop <- w4231 stop-if-true
    # "PID LOGIC"
    n3274 = local read "run test Calibration"() -> (w4219:bool)
    n3275 = local read "RUN"() -> (w4229:bool)
    n3276 = local read "Auto Start Temp"() -> (w4220:bool)
    n3277 = local read "Auto Start Test"() -> (w4228:bool)
    n3278 = local read "START TEMP"() -> (w4218:bool)
    n3279 = And(x=w4220, y=w4228) -> (x .and. y?=w4221:bool)
    n3280 = Or(x=w4229, y=w4221) -> (x .or. y?=w4230:bool)
    n3281 = And(x=w4230, y=w4218) -> (x .and. y?=w4217:bool)
    n3282 = And(x=w4219, y=w4218) -> (x .and. y?=w4216:bool)
    n3283 = Or(x=w4216, y=w4217) -> (x .or. y?=w4215:bool)
    n3284 = Wait (ms)(milliseconds to wait="milliseconds to wait") -> ()  [unwired: 1 out]
    n3285 = case shown="True" w4215 {
      tunnel: [400.0 ("out_vc_cmd") w4250] -> w4222
      tunnel: [w4234 w4252] -> w4223
      tunnel: [w4234 w4251] -> w4224
      tunnel: w4227 -> [_ w4241]
      tunnel: w4226 -> [_ w4240]
      tunnel: w4225 -> [_ w4239]
      tunnel: w4219 -> [_ w4235]
      frame False {
        w4234 = 0.0 ("error_out")
      }
      frame True {
        n3286 = case shown="True" w4235 {
          tunnel: [w4259 1.0] -> w4237
          frame False {
            n3287 = local read "Set Strk"() -> (w4258:dbl)
            n3288 = Add(x=w4258, y="Add up Stroke") -> (x+y=w4259:dbl)
          }
          frame True {
          }
        }
        n3289 = local read "LVDT STROKE"() -> (w4236:dbl)
        n3290 = formula code="// Zero-Hardcode Explicit Positional-Form PID Engine\n// Inputs: target_stroke, measured_stroke, dt, prev_error, integral_accumulator_in, prev_vc_cmd\n//         kp, ki, kd, max_step_change, max_amplitude, min_amplitude, startup_cmd\n// Outputs: vc_cmd, error_out, out_error, integral_accumulator_out, out_vc_cmd\n\n// 1. Calculate Tracking Error\nfloat current_error = target_stroke - measured_stroke;\nerror_out = current_error;\n\n// 2. Compute Proportional Term\nfloat p_term = kp * current_error;\n\n// 3. Compute Derivative Term\nfloat d_term = 0.0;\nif (dt > 0.0) {\n    d_term = kd * ((current_error - prev_error) / dt);\n}\n\n// 4. Update and Accumulate Integral Term\nfloat current_integral = integral_accumulator_in + (current_error * dt);\nfloat i_term = ki * current_integral;\n\n// 5. Calculate Ideal Target Command (Anchored by startup baseline)\nfloat ideal_command = startup_cmd + p_term + i_term + d_term;\n\n// 6. Apply Loop Rate Limiting FIRST \n// (Forces the command to climb gradually from prev_vc_cmd instead of jumping straight to max)\nfloat raw_adjustment = ideal_command - prev_vc_cmd;\n\nif (raw_adjustment > max_step_change) {\n    raw_adjustment = max_step_change;\n} else if (raw_adjustment < -max_step_change) {\n    raw_adjustment = -max_step_change;\n}\n\nfloat next_vc_cmd = prev_vc_cmd + raw_adjustment;\n\n// 7. Anti-Windup Protection & Final Output Safety Safeguard Clamping\n// (Back-calculating based on what we are ACTUALLY outputting)\nif (next_vc_cmd > max_amplitude) {\n    float excess = next_vc_cmd - max_amplitude;\n    if (ki > 0.0) {\n        current_integral -= excess / ki;\n    }\n    next_vc_cmd = max_amplitude;\n} else if (next_vc_cmd < min_amplitude) {\n    float excess = next_vc_cmd - min_amplitude;\n    if (ki > 0.0) {\n        current_integral -= excess / ki;\n    }\n    next_vc_cmd = min_amplitude;\n}\n\n// 8. Map to Shift Registers for memory persistence\nvc_cmd = next_vc_cmd;\nout_error = current_error;                   \nintegral_accumulator_out = current_integral;  \nout_vc_cmd = next_vc_cmd;"("target_stroke"=w4237, "measured_stroke"=w4236, "dt"="dt", "integral_accumulator_in"=w4240, "prev_error"=w4241, "prev_vc_cmd"=w4239, "kp"="kp", "ki"="ki", "kd"="kd", "max_step_change"="max_step_change", "max_amplitude"="max_amplitude", "min_amplitude"="min_amplitude", "startup_cmd"="startup_cmd") -> ("vc_cmd"=w4256:dbl, "out_error"=w4251:dbl, "integral_accumulator_out"=w4252:dbl, "out_vc_cmd"=w4250:dbl)  [unwired: 1 out]
        "output Vpp" <- w4256
        n3291 = Number To Fractional String(number=w4256, precision (6)=i16 1) -> (F-format string=w4254:string)  [unwired: 2 in]
        n3292 = Concatenate Strings("DAC;" ("string"), w4254) -> (w4238:string)
        n3293 = local write "Due Write"(w4238) -> ()
        "prev_error" <- w4241
        "integral_accumulator_in" <- w4240
        "prev_vc_cmd" <- w4239
      }
    }
    n3294 = local read "Quit"() -> (w4231:bool)
  }
  n3295 = Or(x=w50, y=w49) -> (x .or. y?=w51:bool)
  n3296 = Or(x=w47, y=w51) -> (x .or. y?=w56:bool)
  n3297 = control-ref of="new picture"() -> ()  [unwired: 1 out]
  n3298 = Or(x=w59, y=w56) -> (x .or. y?=w53:bool)
  n3299 = Or(x=w53, y=w54) -> (x .or. y?=w48:bool)
  n3300 = while {
    tunnel: [w4261] -> w58
    i -> [w4268]
    stop <- w4261 stop-if-true
    n3301 = local read "Quit"() -> (w4261:bool)
    n3302 = Equal To 0?(x=w4268) -> (x = 0?=w4266:bool)
    n3303 = call "Elapsed Time3"("Time Target (s)"=45.0, "Auto Reset"=TRUE) -> ("Time has Elapsed"=w4265:bool)  [unwired: 10 in, 7 out]
    n3304 = Wait (ms)(milliseconds to wait=u32 50) -> ()  [unwired: 1 out]
    n3305 = Or(x=w4265, y=w4266) -> (x .or. y?=w4267:bool)
    n3306 = case shown="True" w4267 {
      frame False {
      }
      frame True {
        n3307 = call <vilib>:"System Exec.vi"("run minimized? (F)"=TRUE, "error in (no error)"="error in (no error)", "command line"="powercfg.exe -change -monitor-timeout-ac 0") -> ("error out"=w4279:errorcluster)  [unwired: 5 in, 3 out]
        n3308 = call <vilib>:"System Exec.vi"("run minimized? (F)"=TRUE, "error in (no error)"=w4279, "command line"="powercfg.exe -change -disk-timeout-ac 0") -> ("error out"=w4278:errorcluster)  [unwired: 5 in, 3 out]
        n3309 = call <vilib>:"System Exec.vi"("run minimized? (F)"=TRUE, "error in (no error)"=w4278, "command line"="powercfg.exe -change -standby-timeout-ac 0") -> ("error out"=w4277:errorcluster)  [unwired: 5 in, 3 out]
        n3310 = call <vilib>:"System Exec.vi"("run minimized? (F)"=TRUE, "error in (no error)"=w4277, "command line"="powercfg.exe -change -hibernate-timeout-ac 0") -> ("error out"=w4276:errorcluster)  [unwired: 5 in, 3 out]
        n3311 = call <vilib>:"Simple Error Handler.vi"("error in (no error)"=w4276) -> ("error out"=w4282:errorcluster)  [unwired: 4 in, 4 out]
        n3312 = call <vilib>:"Clear Errors.vi"("error in (no error)"=w4282) -> ("error out"=→"error out":errorcluster)  [unwired: 5 in, 1 out]
      }
    }
  }
  n3313 = Compound Arithmetic op=OR(w61, w48, w58) -> (w60:bool)
  n3314 = flat-sequence {
    tunnel: w60 -> [_]
    tunnel: [w4284] -> w30
    tunnel: w30 -> [_]
    frame #0 {
      n3315 = call "CLOSE CONNECTION.vi"() -> ("error out"=w4284:errorcluster)  [unwired: 11 in]
    }
    frame #1 {
      n3316 = Quit LabVIEW(quit? (T)=TRUE) -> ()
      n3317 = local write "Quit"(FALSE ("EXIT")) -> ()
    }
  }
  n3318 = property on="Heater Button" class="Bool (strict)"("Visible"=TRUE) -> ()  [unwired: 2 in, 2 out]
  n3319 = while {
    tunnel: [w4291] -> _
    i -> [w4291]
    stop <- w4287 stop-if-true
    # "Langauage selection"
    n3320 = Equal?(x="Lan flag", y=22.0) -> ()  [unwired: 1 out]
    n3321 = disable-structure shown="Disabled" {
      frame Disabled {
        n3322 = stacked-sequence {
          frame #0 {
            n3323 = case shown="\"Russian\"" "Language Selection" {
              tunnel: [0 1] -> w4293
              frame "English", Default {
              }
              frame "Russian" {
              }
            }
            n3324 = for {
              N: 130 -> [_]
              tunnel: "Table" -> [w4302]
              tunnel: w4293 -> [w4301]
              i -> [w4300]
              n3325 = Index Array(array=w4302, index (row)=w4300, index (col)=w4301) -> (element=w4299:string)
              n3326 = case shown="1" w4300 {
                tunnel: w4299 -> [w4303 w4304 _ w4305 w4306 w4307 w4308 w4309 w4310 w4311 w4312 w4313 w4314 w4315 w4316 w4317 w4318 w4319 w4320 w4321 w4322 w4323 w4324 w4325 w4326 w4327 w4328 w4329 w4330 _ _ w4331 w4332 w4333 w4334 w4335 w4336 w4345 w4352 w4359 w4366 w4370 w4373 w4376 w4378 w4380 w4381 w4382 w4383 w4384 w4385 w4386 w4387 w4388 w4389 w4390 w4391 w4392 w4393 w4394 w4395 w4396 w4397 w4398 w4399 w4400 w4401 w4402 w4403 w4404 w4405 w4406 w4407 w4408 w4409 w4410 w4411 w4412 w4413 w4414 w4415 w4416 w4417 w4418 w4419 w4420 w4421 w4422 w4423 w4424 w4425 w4426 w4427 w4428 w4429 w4430 w4431 w4432 w4433 w4434 w4435 w4436 w4437 w4438 w4439 _ w4440 w4441 w4442 w4443 w4444 w4445 w4446 w4447 w4448 w4449 w4450 w4451 w4452 _ w4453 w4454 w4455 w4456 w4457 w4458 _]
                frame 0 {
                  n3327 = local write "S"(w4303) -> ()
                }
                frame 1 {
                  n3328 = local write "S 2"(w4304) -> ()
                }
                frame 2 {
                }
                frame 3 {
                  n3329 = local write "S 4"(w4305) -> ()
                }
                frame 4 {
                  n3330 = property on="FILE" class="Str"("Caption.Text"=w4306) -> ()  [unwired: 2 in, 2 out]
                }
                frame 5 {
                  n3331 = property on="Fuel Discription :" class="Str"("Caption.Text"=w4307) -> ()  [unwired: 2 in, 2 out]
                }
                frame 6 {
                  n3332 = property on="Remarks :" class="Str"("Caption.Text"=w4308) -> ()  [unwired: 2 in, 2 out]
                }
                frame 7 {
                  n3333 = property on="Save & Continue" class="Bool (strict)"("Boolean Text.Text"=w4309) -> ()  [unwired: 2 in, 2 out]
                }
                frame 8 {
                }
                frame 9 {
                  n3334 = property on="Set Hz" class="DigNum (strict)"("Caption.Text"=w4311) -> ()  [unwired: 2 in, 2 out]
                }
                frame 10 {
                }
                frame 11 {
                  n3335 = property on="NORMAL LOAD" class="DigNum (strict)"("Caption.Text"=w4313) -> ()  [unwired: 2 in, 2 out]
                }
                frame 12 {
                }
                frame 13 {
                  n3336 = property on="Set Temp" class="DigNum (strict)"("Caption.Text"=w4315) -> ()  [unwired: 2 in, 2 out]
                }
                frame 14 {
                  n3337 = local write "S 15"(w4316) -> ()
                }
                frame 15 {
                  n3338 = property on="Set Rh" class="DigNum (strict)"("Caption.Text"=w4317) -> ()  [unwired: 2 in, 2 out]
                }
                frame 16 {
                }
                frame 17 {
                  n3339 = local write "S 18"(w4319) -> ()
                }
                frame 18 {
                  "String 17" <- w4320
                }
                frame 19 {
                  n3340 = property on="test time" class="DigNum (strict)"("Caption.Text"=w4321) -> ()  [unwired: 2 in, 2 out]
                }
                frame 20 {
                  "String 18" <- w4322
                  "String 22" <- w4322
                }
                frame 21 {
                  n3341 = property on="Elapsed time" class="DigNum (strict)"("Caption.Text"=w4323) -> ()  [unwired: 2 in, 2 out]
                }
                frame 22 {
                  n3342 = property on="Samplingtime 2" class="DigNum (strict)"("Caption.Text"=w4324) -> ()  [unwired: 2 in, 2 out]
                }
                frame 23 {
                  "String 21" <- w4325
                }
                frame 24 {
                  n3343 = property on="Countdown" class="DigNum (strict)"("Caption.Text"=w4326) -> ()  [unwired: 2 in, 2 out]
                }
                frame 25 {
                  n3344 = property on="Countdown 2" class="DigNum (strict)"("Caption.Text"=w4327) -> ()  [unwired: 2 in, 2 out]
                }
                frame 26 {
                  n3345 = property on="Engage" class="Bool (strict)"("Boolean Text.Text"=w4328) -> ()  [unwired: 2 in, 2 out]
                }
                frame 27 {
                  n3346 = property on="Boolean  4" class="Bool (strict)"("Boolean Text.Text"=w4329) -> ()  [unwired: 2 in, 2 out]
                }
                frame 28 {
                  n3347 = property on="Test \nStatus" class="Bool (strict)"("Boolean Text.Text"=w4330) -> ()  [unwired: 2 in, 2 out]
                }
                frame 29 {
                }
                frame 30 {
                }
                frame 31 {
                }
                frame 32 {
                  n3348 = property on="RSTCOF" class="Bool"("Boolean Text.Text"=w4332) -> ()  [unwired: 2 in, 2 out]
                  n3349 = property on="RST FF" class="Bool"("Boolean Text.Text"=w4332) -> ()  [unwired: 2 in, 2 out]
                  n3350 = property on="RST TEMP" class="Bool"("Boolean Text.Text"=w4332) -> ()  [unwired: 2 in, 2 out]
                  n3351 = property on="RSTV1 3" class="Bool"("Boolean Text.Text"=w4332) -> ()  [unwired: 2 in, 2 out]
                  n3352 = property on="rstv2" class="Bool"("Boolean Text.Text"=w4332) -> ()  [unwired: 2 in, 2 out]
                  n3353 = property on="RSTV1 2" class="Bool"("Boolean Text.Text"=w4332) -> ()  [unwired: 2 in, 2 out]
                  n3354 = property on="RST CP" class="Bool"("Boolean Text.Text"=w4332) -> ()  [unwired: 2 in, 2 out]
                }
                frame 33 {
                  "S 61" <- w4333
                }
                frame 34 {
                  "String 23" <- w4334
                }
                frame 35 {
                  n3355 = property on="Rh Before" class="DigNum (strict)"("Caption.Text"=w4335) -> ()  [unwired: 2 in, 2 out]
                }
                frame 36 {
                  n3356 = Match Pattern(string=w4336, regular expression=",") -> (before substring=→"bs":string, after substring=→"as":string)  [unwired: 1 in, 2 out]
                  n3357 = property on="Rh After" class="DigNum (strict)"("Caption.Text"=w4336) -> ()  [unwired: 2 in, 2 out]
                }
                frame 37 {
                  n3358 = Match Pattern(string=w4345, regular expression=",") -> (before substring=w4344:string, after substring=w4343:string)  [unwired: 1 in, 2 out]
                  "bs" <- w4344
                  "as" <- w4343
                  n3359 = Concatenate Strings(w4344, w4343) -> (w4340:string)
                  n3360 = property on="Humidity before test 2" class="DigNum (strict)"("Caption.Text"=w4340) -> ()  [unwired: 2 in, 2 out]
                  n3361 = Concatenate Strings(w4340, "=" ("string")) -> (w4341:string)
                  n3362 = local write "S 38"(w4341) -> ()
                }
                frame 38 {
                  n3363 = Match Pattern(string=w4352, regular expression=",") -> (before substring=w4351:string, after substring=w4350:string)  [unwired: 1 in, 2 out]
                  "bs" <- w4351
                  "as" <- w4350
                  n3364 = Concatenate Strings(w4351, w4350) -> (w4347:string)
                  n3365 = property on="Humidity after test 2" class="DigNum (strict)"("Caption.Text"=w4347) -> ()  [unwired: 2 in, 2 out]
                  n3366 = Concatenate Strings(w4347, "=" ("string")) -> (w4349:string)
                  n3367 = local write "S 39"(w4349) -> ()
                }
                frame 39 {
                  n3368 = Match Pattern(string=w4359, regular expression=",") -> (before substring=w4358:string, after substring=w4357:string)  [unwired: 1 in, 2 out]
                  "bs" <- w4358
                  "as" <- w4357
                  n3369 = Concatenate Strings(w4358, w4357) -> (w4354:string)
                  n3370 = property on="Temperature before test 2" class="DigNum (strict)"("Caption.Text"=w4354) -> ()  [unwired: 2 in, 2 out]
                  n3371 = Concatenate Strings(w4354, "=" ("string")) -> (→"String 34":string)
                }
                frame 40 {
                  n3372 = Match Pattern(string=w4366, regular expression=",") -> (before substring=w4365:string, after substring=w4364:string)  [unwired: 1 in, 2 out]
                  "bs" <- w4365
                  "as" <- w4364
                  n3373 = Concatenate Strings(w4365, w4364) -> (w4361:string)
                  n3374 = property on="Temperature after test 2" class="DigNum (strict)"("Caption.Text"=w4361) -> ()  [unwired: 2 in, 2 out]
                  n3375 = Concatenate Strings(w4361, "=" ("string")) -> (→"String 35":string)
                  n3376 = property on="Temperature after test" class="DigNum (strict)"("Caption.Text"=w4361) -> ()  [unwired: 2 in, 2 out]
                }
                frame 41 {
                  n3377 = property on="AVP 2" class="DigNum (strict)"("Caption.Text"=w4370) -> ()  [unwired: 2 in, 2 out]
                  n3378 = Concatenate Strings(w4370, "=" ("string")) -> (→"String 36":string)
                }
                frame 42 {
                  n3379 = property on="MWSD 2" class="DigNum (strict)"("Caption.Text"=w4373) -> ()  [unwired: 2 in, 2 out]
                  n3380 = Concatenate Strings(w4373, "=" ("string")) -> (→"String 37":string)
                }
                frame 43 {
                  n3381 = property on="HCF 2" class="DigNum (strict)"("Caption.Text"=w4376) -> ()  [unwired: 2 in, 2 out]
                  n3382 = Concatenate Strings(w4376, "=" ("string")) -> (→"String 38":string)
                }
                frame 44 {
                  n3383 = Concatenate Strings(w4378, "=" ("string")) -> (→"String 39":string)
                  n3384 = property on="WS1.4 2" class="DigNum (strict)"("Caption.Text"=w4378) -> ()  [unwired: 2 in, 2 out]
                }
                frame 45 {
                }
                frame 46 {
                  n3385 = local write "S 47"(w4381) -> ()
                }
                frame 47 {
                  n3386 = local write "S 48"(w4382) -> ()
                }
                frame 48 {
                  n3387 = local write "S 49"(w4383) -> ()
                }
                frame 49 {
                  n3388 = local write "S 50"(w4384) -> ()
                }
                frame 50 {
                  n3389 = local write "S 51"(w4385) -> ()
                }
                frame 51 {
                  n3390 = local write "S 52"(w4386) -> ()
                }
                frame 52 {
